vi "8.8.2.vi"() -> ()   [LabVIEW 2018]
panel:
  in  "정지":bool
  out "a":dbl(graph)
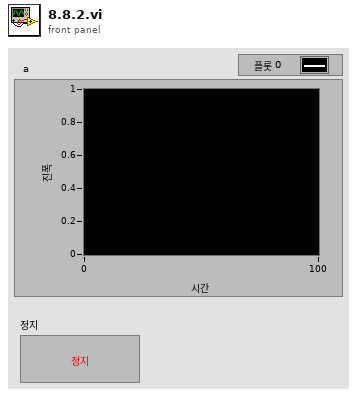
[diagram p1: front panel]
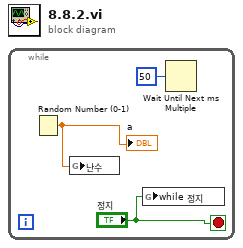
[diagram p0: block diagram]
diagram:
  n1 = while {
    stop <- "정지" stop-if-true
    n2 = Random Number (0-1)() -> (number: 0 to 1=w2:dbl)
    "a" <- w2
    n3 = global write "8.8.2_글로벌.vi" "난수"(w2) -> ()
    n4 = global write "8.8.2_글로벌.vi" "while 정지"("정지") -> ()
    n5 = Wait Until Next ms Multiple(millisecond multiple=u32 50 ("ms 배수")) -> ()  [unwired: 1 out]
  }
